vi "Main.vi"() -> ()   [LabVIEW 2018]
panel:
  in  "View Type":i32(listbox)
  out "error out":errorcluster
  in  "stop":bool
  in  "Tree":string[](tree)
  out "output cluster":T1
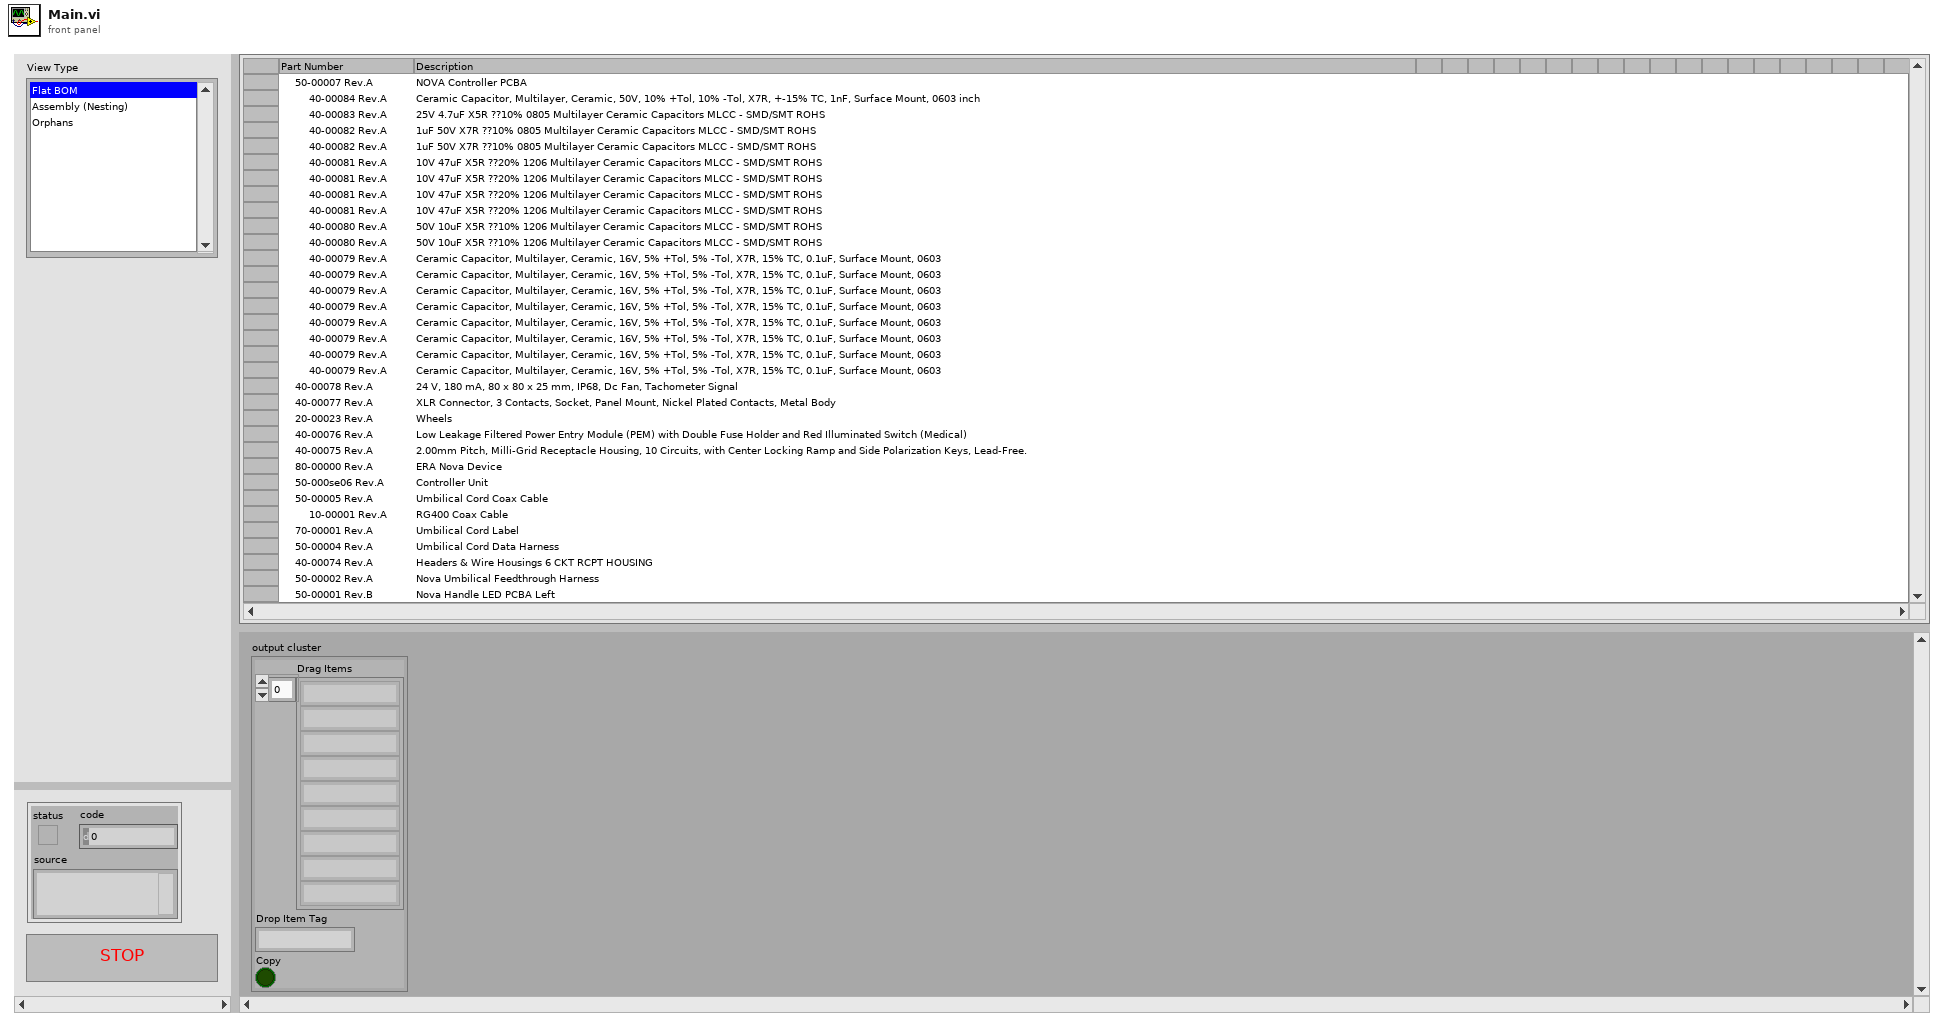
[diagram p1: front panel]
types:
  T1 = cluster{"Drag Items":string[], "Drop Item Tag":string, "Copy":bool}
  T2 = cluster{"Drag Items Tags":string[], "Drop Item Tag":string, "Copy":bool}
  T3 = enum8{"Enabled", "Disabled", "Disabled and Grayed Out"}
  T4 = cluster{"data name":string, "drag data":variant}[]
  T5 = typedef "LVPoint32TypeDef.ctl" = cluster{"Horizontal":i32, "Vertical":i32}
  T6 = cluster{"Shift":bool, "Ctrl":bool, "Alt":bool, "Cmd":bool, "Opt":bool}
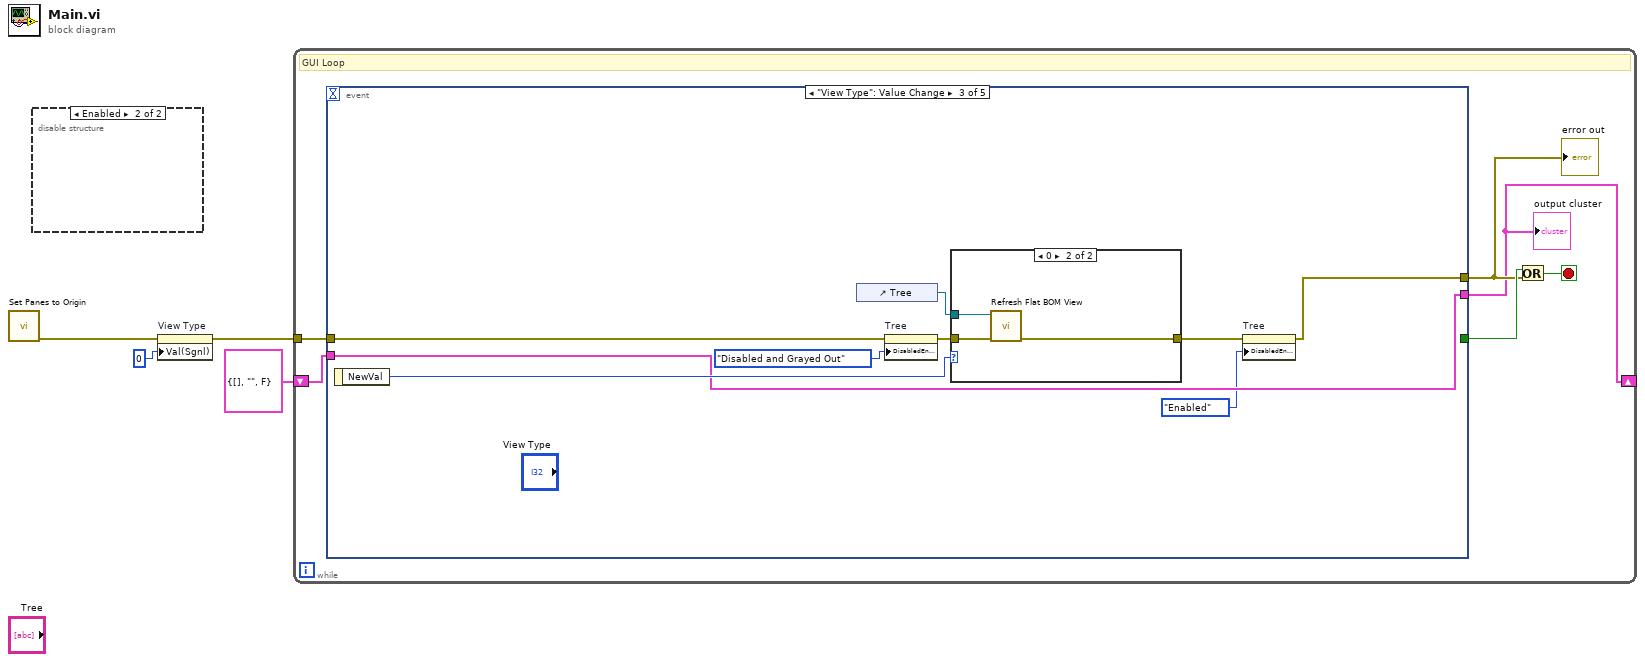
[diagram p0: block diagram]
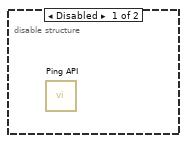
[diagram p2: hidden frame]
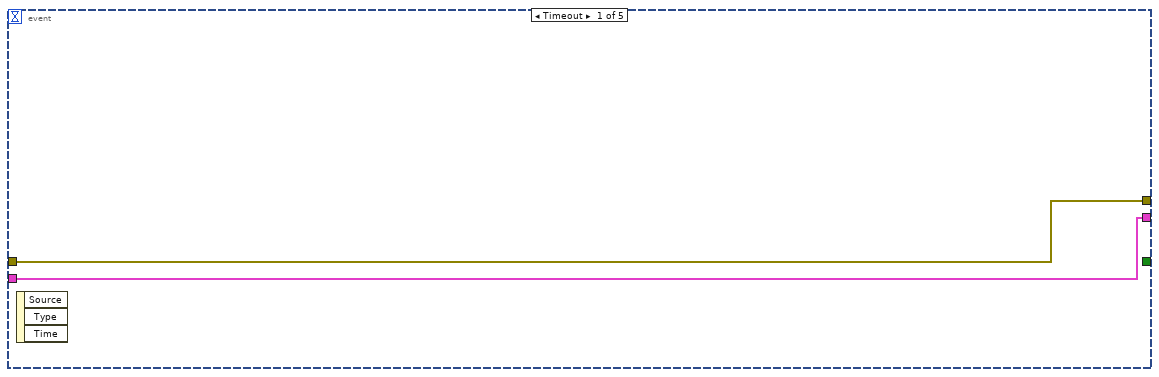
[diagram p3: hidden frame]
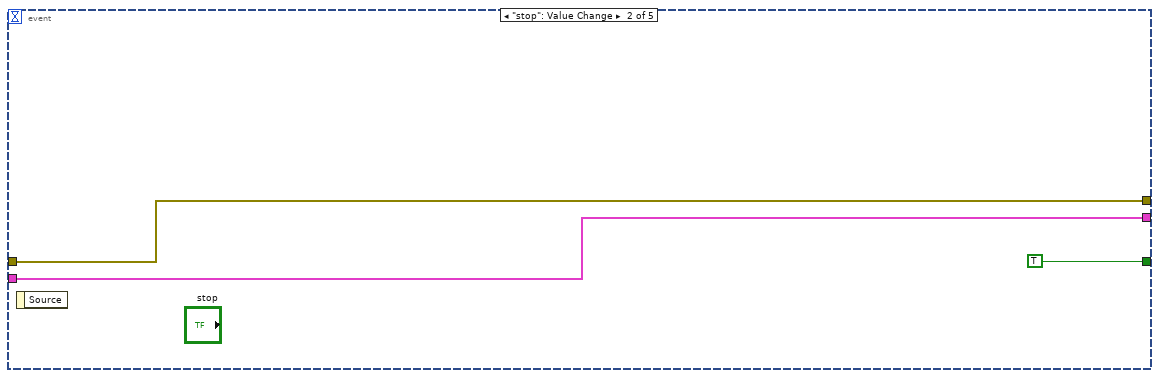
[diagram p4: hidden frame]
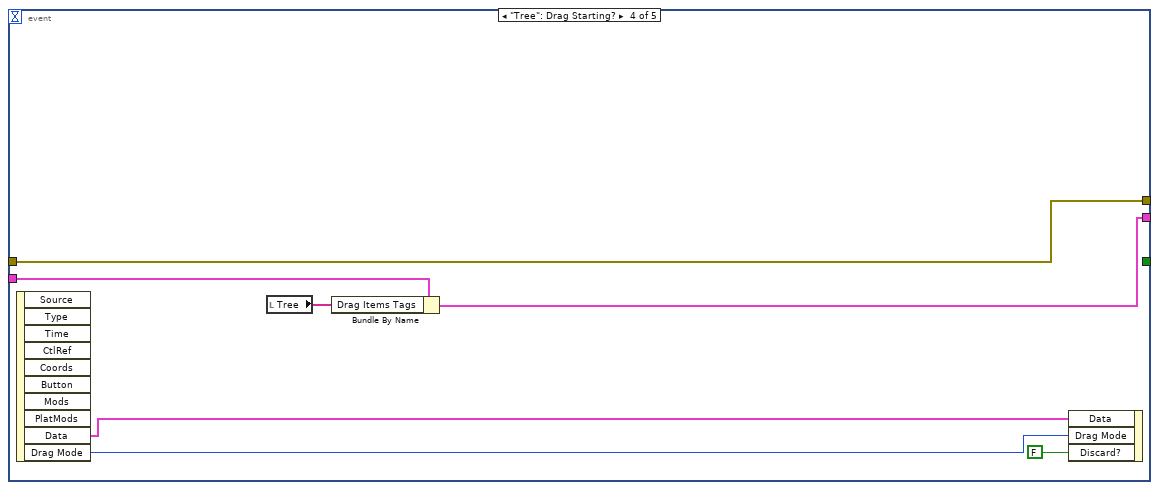
[diagram p6: hidden frame]
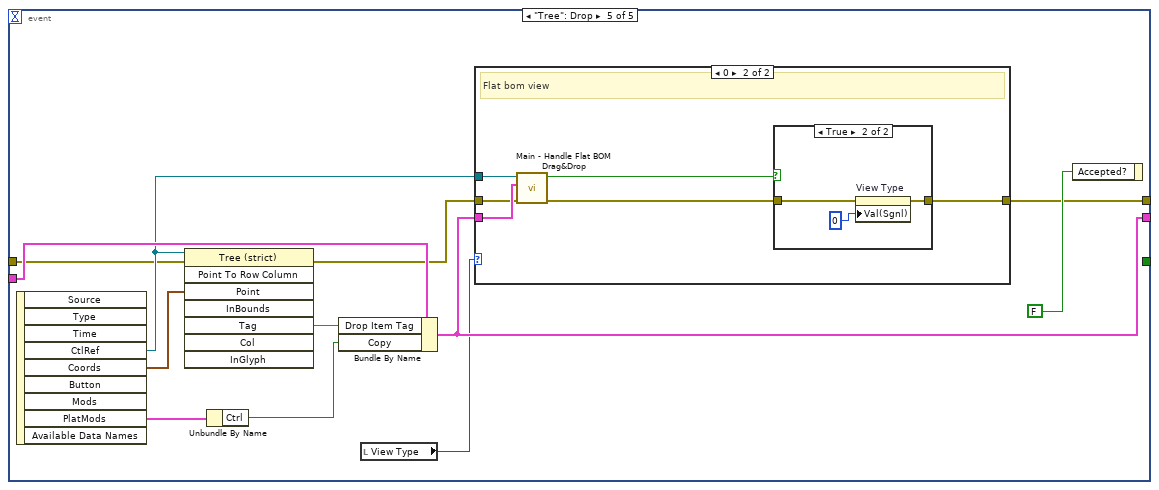
[diagram p7: hidden frame]
diagram:
  n1 = call "Set Panes to Origin.vi"() -> ("Error out"=w3:errorcluster)  [unwired: 11 in]
  n2 = disable-structure shown="Enabled" {
    frame Disabled {
      n3 = call "Ping API.vi"() -> ()  [unwired: 10 in, 2 out]
    }
    frame Enabled {
    }
  }
  n4 = property on="View Type" class="LstBox (strict)"(error in=w3, "Val(Sgnl)"=0 ("Value (Signaling)")) -> (error out=w1:errorcluster)  [unwired: 1 in, 1 out]
  n5 = while {
    shift-right: [w7] -> _
    shift-left: T2 {"Drag Items Tags"=[], "Drop Item Tag"="", "Copy"=FALSE} ("output cluster") -> [w6]
    tunnel: w1 -> [w5]
    stop <- w9 stop-if-true
    # "GUI Loop"
    n6 = event shown="[2] \"View Type\": Value Change" {
      selector: _ -> [_ _ _ _ _]
      dyn-events: _ -> [_ _ _ _ _]
      timeout: _ -> [_ _ _ _ _]
      tunnel: [_ TRUE _ _ _] -> w10
      tunnel: [w11 w13 w19 w29 w41] -> w8
      tunnel: [w12 w14 w22 w31 w40] -> w7
      tunnel: w6 -> [w12 w14 w22 w30 w47]
      tunnel: w5 -> [w11 w13 w16 w29 w36]
      event Timeout {
        n7 = event-data() -> ()  [unwired: 1 in, 3 out]
      }
      event "stop": Value Change {
        n8 = event-data() -> ()  [unwired: 1 in, 1 out]
      }
      event "View Type": Value Change {
        n9 = event-data() -> ("NewVal"=w24:i32)  [unwired: 1 in]
        n10 = control-ref of="Tree"() -> (w23:refnum<vi>)
        n11 = property on="Tree" class="Tree (strict)"(error in=w16, "DisabledEnum"=T3."Disabled and Grayed Out" ("Disabled")) -> (error out=w21:errorcluster)  [unwired: 1 in, 1 out]
        n12 = case shown="0" w24 {
          tunnel: [w25 w28] -> w20
          tunnel: w23 -> [_ w27]
          tunnel: w21 -> [w25 w26]
          frame Default {
          }
          frame 0 {
            n13 = call "Refresh Flat BOM View.vi"("Error in"=w26, "Tree"=w27) -> ("Error out"=w28:errorcluster)  [unwired: 9 in]
          }
        }
        n14 = property on="Tree" class="Tree (strict)"(error in=w20, "DisabledEnum"=T3."Enabled" ("Disabled")) -> (error out=w19:errorcluster)  [unwired: 1 in, 1 out]
      }
      event "Tree": Drag Starting? {
        n15 = event-data() -> ("Data"=w34:T4, "Drag Mode"=w35:enum32{"copy or move", "copy only", "move only"})  [unwired: 1 in, 8 out]
        n16 = local read "Tree"() -> (w32:string[])
        n17 = Bundle By Name(cluster=w30, "Drag Items Tags"=w32) -> (w31:T2)
        n18 = event-data("Data"=w34, "Drag Mode"=w35, "Discard?"=FALSE) -> ()  [unwired: 1 in, 1 out]
      }
      event "Tree": Drop {
        n19 = event-data() -> ("CtlRef"=w39:refnum<vi>, "Coords"=w46:T5, "PlatMods"=w43:T6)  [unwired: 1 in, 6 out]
        n20 = invoke class="Tree (strict)" method="Point To Row Column"(reference=w39, error in=w36, "Point"=w46) -> (error out=w37:errorcluster, "Tag"=w45:string)  [unwired: 5 in, 6 out]
        n21 = Unbundle By Name(w43) -> ("Ctrl"=w42:bool)
        n22 = Bundle By Name(cluster=w47, "Drop Item Tag"=w45, "Copy"=w42) -> (w40:T2)
        n23 = local read "View Type"() -> (w38:i32)
        n24 = case shown="0" w38 {
          tunnel: [w48 w50] -> w41
          tunnel: w40 -> [_ w54]
          tunnel: w39 -> [_ w53]
          tunnel: w37 -> [w48 w51]
          frame Default {
          }
          frame 0 {
            # "Flat bom view"
            n25 = call "Main - Handle Flat BOM Drag&Drop.vi"("error in (no error)"=w51, "Drag&Drop Data"=w54, "TreeControl in"=w53) -> ("error out"=w49:errorcluster, "Refresh Table"=w52:bool)  [unwired: 6 in, 1 out]
            n26 = case shown="True" w52 {
              tunnel: w49 -> [w55 w57]
              tunnel: [w55 w56] -> w50
              frame False {
                # "Don't refresh the table"
              }
              frame True {
                n27 = property on="View Type" class="LstBox (strict)"(error in=w57, "Val(Sgnl)"=0 ("Value (Signaling)")) -> (error out=w56:errorcluster)  [unwired: 1 in, 1 out]
              }
            }
          }
        }
        n28 = event-data("Accepted?"=FALSE) -> ()  [unwired: 1 in, 1 out]
      }
    }
    "error out" <- w8
    "output cluster" <- w7
    n29 = Or(x=w10, y=w8) -> (x .or. y?=w9:bool)
  }
